vi "Grid_Init_v4.vi"(6 "Part of multigrid":bool, 7 "resume":T1, 8 "Error in":errorcluster, 10 "Settings":T2={"Drift Correction Settings"={"Drift Correction every"=80, "Drift correction Pixels"=256, "Channel index (0-23)"=0, "MaxImagesBack"=2, "Threshold"=2, "Increment"=8, "max applied Drift Correction"=20, "Correct Drift"=TRUE, "Correlate"=0, "Correct z drift"=FALSE, "zdrift \nDuration (s)"=0.0}, "Spectroscopy Setting"={"Imaging Current"=1e-11, "ref Current"=7e-11, "tip Speed (m/s)"=2e-09, "Imaging Bias"=0.02, "ref Bias"=-0.1, "preSTS delay [ms]"=500, "STS z offset"=2e-10, "during Spec Bias (V)"=-0.1, "trigger1 < Hz"=0.0, "trigger 2 >Hz"=0.0, "autoStop"=FALSE, "Spectroscopy"=0, "PLL ON/OFF"=TRUE, "readjust setpoint every "=1, "z Reference"=FALSE, "Lock In"=TRUE}, "Misc"={"File name"="symmetric_node_zOff=200p", "Email when finished"="cornelius.krull@monash.edu,Dhaneesh.Gopalakrishnan@monash.edu,marina.castelli@monash.edu"}, "Grid Settings"={"type"=1, "type order"=1, "X pixel"=0, "Y pixel"=0, "Grid_Parms"={"center X (m)"=0.0, "center Y (m)"=0.0, "width (m)"=0.0, "height (m)"=0.0, "angle (deg)"=0.0}}} {"Grid Settings"."type order" items=["Line", "Grid"]; "Grid Settings"."type" items=["Line", "Grid"]; "Spectroscopy Setting"."Spectroscopy" items=["Bias", "zSpec"]; "Spectroscopy Setting"."trigger 2 >Hz" format="%#_6p"; "Spectroscopy Setting"."trigger1 < Hz" format="%#_6p"; "Spectroscopy Setting"."during Spec Bias (V)" format="%#_5p"; "Spectroscopy Setting"."STS z offset" format="%#_6p"; "Spectroscopy Setting"."ref Bias" format="%#_6p"; "Spectroscopy Setting"."Imaging Bias" format="%#_6p"; "Spectroscopy Setting"."tip Speed (m/s)" format="%.2p"; "Spectroscopy Setting"."ref Current" format="%#_6p"; "Spectroscopy Setting"."Imaging Current" format="%#_6p"; "Drift Correction Settings"."Correlate" items=["first Frame", "successive Frames"]; "Drift Correction Settings"."max applied Drift Correction" min=1 max=100 step=1 format="%.0p"; "Drift Correction Settings"."Threshold" min=1 step=1; "Drift Correction Settings"."Channel index (0-23)" items=["Current"=0, "Z (m)"=14]}, 11 "Application reference":refnum<vi>) -> (0 "error out":errorcluster, 1 "FileRefs":T3, 2 "Settings out":T2={"Drift Correction Settings"={"Drift Correction every"=80, "Drift correction Pixels"=256, "Channel index (0-23)"=0, "MaxImagesBack"=2, "Threshold"=2, "Increment"=8, "max applied Drift Correction"=20, "Correct Drift"=TRUE, "Correlate"=0, "Correct z drift"=FALSE, "zdrift \nDuration (s)"=0.0}, "Spectroscopy Setting"={"Imaging Current"=1e-11, "ref Current"=7e-11, "tip Speed (m/s)"=2e-09, "Imaging Bias"=0.02, "ref Bias"=-0.1, "preSTS delay [ms]"=500, "STS z offset"=2e-10, "during Spec Bias (V)"=-0.1, "trigger1 < Hz"=0.0, "trigger 2 >Hz"=0.0, "autoStop"=FALSE, "Spectroscopy"=0, "PLL ON/OFF"=TRUE, "readjust setpoint every "=1, "z Reference"=FALSE, "Lock In"=TRUE}, "Misc"={"File name"="symmetric_node_zOff=200p", "Email when finished"="cornelius.krull@monash.edu,Dhaneesh.Gopalakrishnan@monash.edu,marina.castelli@monash.edu"}, "Grid Settings"={"type"=1, "type order"=1, "X pixel"=0, "Y pixel"=0, "Grid_Parms"={"center X (m)"=0.0, "center Y (m)"=0.0, "width (m)"=0.0, "height (m)"=0.0, "angle (deg)"=0.0}}} caption="Settings" {"Grid Settings"."type order" items=["Line", "Grid"]; "Grid Settings"."type" items=["Line", "Grid"]; "Spectroscopy Setting"."Spectroscopy" items=["Bias", "zSpec"]; "Spectroscopy Setting"."trigger 2 >Hz" format="%#_6p"; "Spectroscopy Setting"."trigger1 < Hz" format="%#_6p"; "Spectroscopy Setting"."during Spec Bias (V)" format="%#_5p"; "Spectroscopy Setting"."STS z offset" format="%#_6p"; "Spectroscopy Setting"."ref Bias" format="%#_6p"; "Spectroscopy Setting"."Imaging Bias" format="%#_6p"; "Spectroscopy Setting"."tip Speed (m/s)" format="%.2p"; "Spectroscopy Setting"."ref Current" format="%#_6p"; "Spectroscopy Setting"."Imaging Current" format="%#_6p"; "Drift Correction Settings"."Correlate" items=["first Frame", "successive Frames"]; "Drift Correction Settings"."max applied Drift Correction" min=1 max=100 step=1 format="%.0p"; "Drift Correction Settings"."Threshold" min=1 step=1; "Drift Correction Settings"."Channel index (0-23)" items=["Current"=0, "Z (m)"=14]}, 3 "Application ref out":refnum<vi>, 5 "DC images":dbl[][][](array[numeric]))   [LabVIEW 2014]
uses:
  <userlib>/Nanonis Prog Interface V5/Nanonis Prog Interface.lvlib
panel:
  # "RUN smart tilt before starting the GRID\nImg Angle = 0  CHECK CUTOFF\nmove tip to reference point for tip height"
  # "z Spectroscopy"
  # "GRID points"
  # "Increase this if no Drift was detected for \na certain number of images"
  # "% of image size"
  # "RUN smart tilt before starting the GRID\nImg Angle = 0  CHECK CUTOFF\nmove tip to reference point for tip height"
  # "z Spectroscopy"
  # "GRID points"
  # "Increase this if no Drift was detected for \na certain number of images"
  # "% of image size"
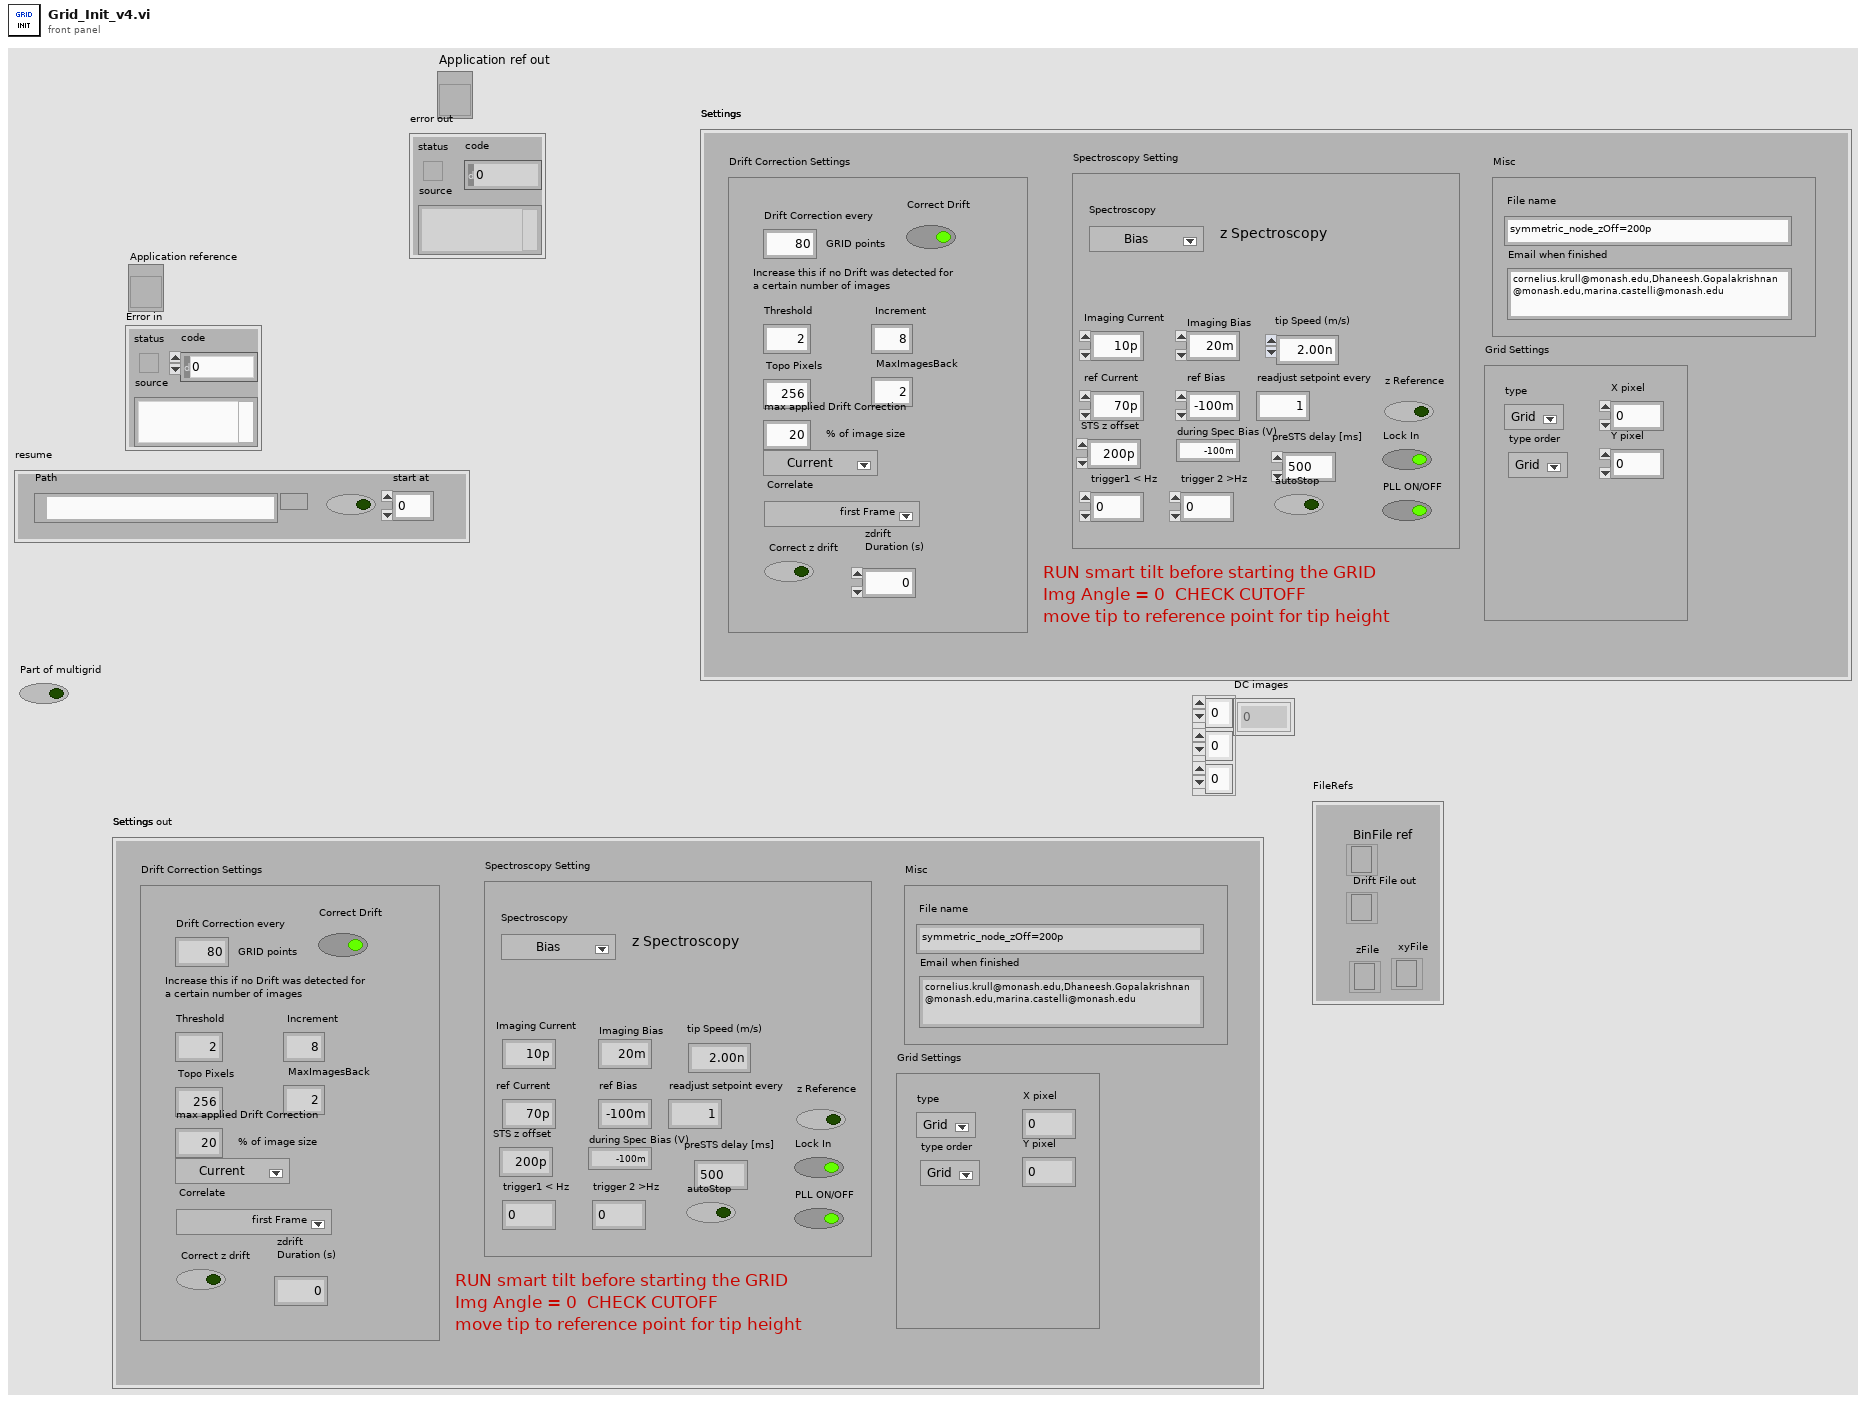
[diagram p1: front panel]
types:
  T1 = cluster{"resume Grid":bool, "Path":path, "start at":i32}
  T2 = cluster{"Drift Correction Settings":cluster{"Drift Correction every":i32, "Drift correction Pixels":i32, "Channel index (0-23)":u8, "MaxImagesBack":i32, "Threshold":i32, "Increment":i32, "max applied Drift Correction":i32, "Correct Drift":bool, "Correlate":u16, "Correct z drift":bool, "zdrift \nDuration (s)":dbl}, "Spectroscopy Setting":cluster{"Imaging Current":dbl, "ref Current":dbl, "tip Speed (m/s)":sgl, "Imaging Bias":dbl, "ref Bias":dbl, "preSTS delay [ms]":u32, "STS z offset":dbl, "during Spec Bias (V)":sgl, "trigger1 < Hz":sgl, "trigger 2 >Hz":sgl, "autoStop":bool, "Spectroscopy":u16, "PLL ON/OFF":bool, "readjust setpoint every ":i32, "z Reference":bool, "Lock In":bool}, "Misc":cluster{"File name":string, "Email when finished":string}, "Grid Settings":cluster{"type":u16, "type order":u16, "X pixel":i32, "Y pixel":i32, "Grid_Parms":cluster{"center X (m)":sgl, "center Y (m)":sgl, "width (m)":sgl, "height (m)":sgl, "angle (deg)":sgl}}}
  T3 = cluster{"Drift File out":refnum<file>, "zFile":refnum<file>, "BinFile ref":refnum<file>, "xyFile":refnum<file>}
  T4 = cluster{"type":u16, "type order":u16, "X pixel":i32, "Y pixel":i32, "Grid_Parms":cluster{"center X (m)":sgl, "center Y (m)":sgl, "width (m)":sgl, "height (m)":sgl, "angle (deg)":sgl}}
  T5 = cluster{"type":u16, "type order":u16, "X pixel":dbl, "Y pixel":dbl, "Grid_Parms":cluster{"center X (m)":sgl, "center Y (m)":sgl, "width (m)":sgl, "height (m)":sgl, "angle (deg)":sgl}}
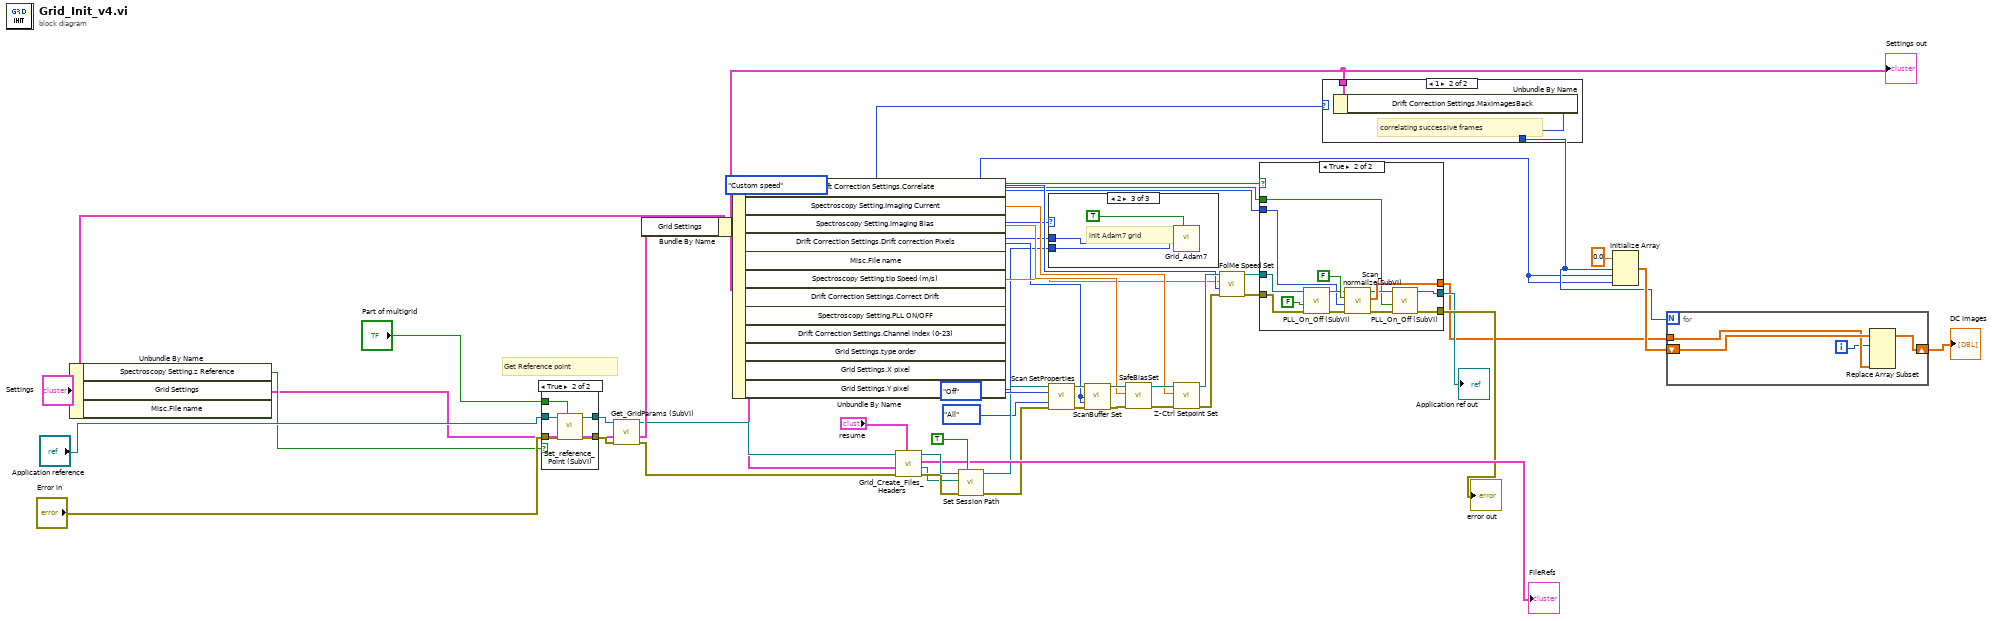
[diagram p0: block diagram]
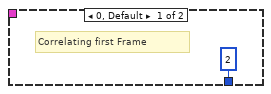
[diagram p4: hidden frame]
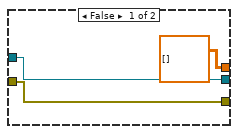
[diagram p5: hidden frame]
diagram:
  # "Get Reference point"
  n1 = Unbundle By Name("Settings") -> ("Spectroscopy Setting.z Reference"=w49:bool, "Grid Settings"=w46:T4)  [unwired: 1 out]
  n2 = case shown="True" w49 {
    tunnel: "Application reference" -> [w53 w58]
    tunnel: "Error in" -> [w52 w57]
    tunnel: [w53 w56] -> w48
    tunnel: [w52 w55] -> w47
    tunnel: "Part of multigrid" -> [_ w54]
    frame False {
    }
    frame True {
      n3 = call "Set_reference_Point (SubVI).vi"("Part of multigrid"=w54, "error in (no error)"=w57, "Application in"=w58) -> ("error out"=w55:errorcluster, "Application out"=w56:refnum<vi>)  [unwired: 7 in]
    }
  }
  n4 = call "Get_GridParams (SubVI).vi"("error in (no error)"=w47, "Grid Settings"=w46, "Application in"=w48) -> ("error out"=w42:errorcluster, "Grid Settings"=w44:T5, "Application out"=w43:refnum<vi>)  [unwired: 5 in, 1 out]
  n5 = Bundle By Name(cluster="Settings", "Grid Settings"=w44) -> (w6:T2)
  "Settings out" <- w6
  n6 = Unbundle By Name(w6) -> ("Drift Correction Settings.Correlate"=w7:u16, "Spectroscopy Setting.Imaging Current"=w26:dbl, "Spectroscopy Setting.Imaging Bias"=w29:dbl, "Drift Correction Settings.Drift correction Pixels"=w8:i32, "Spectroscopy Setting.tip Speed (m/s)"=w22:sgl, "Drift Correction Settings.Correct Drift"=w17:bool, "Spectroscopy Setting.PLL ON/OFF"=w16:bool, "Drift Correction Settings.Channel index (0-23)"=w15:u8, "Grid Settings.type order"=w5:u16, "Grid Settings.X pixel"=w4:i32, "Grid Settings.Y pixel"=w3:i32)  [unwired: 1 out]
  n7 = call "Grid_Create_Files_Headers.vi"("resume"="resume", "Error in (no error)"=w42, "Settings"=w6, "Application ref in"=w43) -> ("error out"=w39:errorcluster, "topoFilePath"=w14:path, "FileRefs"=→"FileRefs":T3, "Application ref out"=w41:refnum<vi>)  [unwired: 4 in]
  n8 = call <userlib>:"Set Session Path.vi"("Save settings to previous? (False)"=TRUE, "error in (no error)"=w39, "Session Folder"=w14, "Application ref in"=w41) -> ("error out"=w33:errorcluster, "Application ref out"=w34:refnum<vi>)  [unwired: 6 in]
  n9 = case shown="2" w5 {
    tunnel: w4 -> [_ _ w60]
    tunnel: w3 -> [_ _ w59]
    frame 0, Default {
    }
    frame 1 {
    }
    frame 2 {
      # "init Adam7 grid"
      n10 = call "Grid_Adam7.vi"("reset"=TRUE, "py 2"=w59, "px 2"=w60) -> ()  [unwired: 7 in, 2 out]
    }
  }
  n11 = call <userlib>:"Scan SetProperties.vi"("Application ref in"=w34, "Continuous scan"=enum16{"No change", "On", "Off"}."Off", "Auto save"=enum16{"No change", "All", "Next", "Off"}."All", "Error in (no error)"=w33) -> ("Application ref out"=w36:refnum<vi>, "Error out"=w35:errorcluster)  [unwired: 10 in]
  n12 = call <userlib>:"ScanBuffer Set.vi"("Application ref in"=w36, "Pixels"=w8, "Lines"=w8, "error in (no error)"=w35) -> ("Application ref out"=w31:refnum<vi>, "error out"=w30:errorcluster)  [unwired: 10 in]
  n13 = call "SafeBiasSet.vi"("Application ref in"=w31, "Bias (V)"=w29, "error in (no error)"=w30) -> ("Application ref out"=w27:refnum<vi>, "Error out"=w28:errorcluster)  [unwired: 6 in]
  n14 = call <userlib>:"Z-Ctrl Setpoint Set.vi"("error in (no error)"=w28, "Z Controller setpoint"=w26, "Application ref in"=w27) -> ("error out"=w24:errorcluster, "Application ref out"=w25:refnum<vi>)  [unwired: 7 in]
  n15 = call <userlib>:"FolMe Speed Set.vi"("error in (no error)"=w24, "Speed Setting (Custom)"=enum32{"Scan speed", "Custom speed"}."Custom speed", "Speed (m/s)"=w22, "Application ref in"=w25) -> ("error out"=w20:errorcluster, "Application ref out"=w21:refnum<vi>)  [unwired: 4 in]
  n16 = case shown="True" w17 {
    tunnel: [dbl[][] [] ("Array") w77] -> w11
    tunnel: w21 -> [w64 w75]
    tunnel: [w64 w71] -> w18
    tunnel: w20 -> [w62 w70]
    tunnel: [w62 w67] -> w19
    tunnel: w16 -> [_ w66]
    tunnel: w15 -> [_ w65]
    frame False {
    }
    frame True {
      n17 = call "PLL_On_Off (SubVI).vi"("error in (no error)"=w70, "Output ON/OFF (F=OFF)"=FALSE, "Application in"=w75) -> ("error out"=w69:errorcluster, "Application out"=w74:refnum<vi>)  [unwired: 7 in]
      n18 = call "Scan_normailze(SubVI).vi"("error in (no error)"=w69, "Channel index (0-23)"=w65, "Normalization"=FALSE ("Boolean"), "Application in"=w74) -> ("error out"=w68:errorcluster, "Array"=w77:dbl[][], "Application out"=w72:refnum<vi>)  [unwired: 5 in]
      n19 = call "PLL_On_Off (SubVI).vi"("error in (no error)"=w68, "Output ON/OFF (F=OFF)"=w66, "Application in"=w72) -> ("error out"=w67:errorcluster, "Application out"=w71:refnum<vi>)  [unwired: 7 in]
    }
  }
  "Application ref out" <- w18
  "error out" <- w19
  n20 = case shown="1" w7 {
    tunnel: w6 -> [_ w80]
    tunnel: [2 ("MaxImagesBack") w79] -> w10
    frame 0, Default {
      # "Correlating first Frame"
    }
    frame 1 {
      # "correlating successive frames"
      n21 = Unbundle By Name(w80) -> ("Drift Correction Settings.MaxImagesBack"=w79:i32)
    }
  }
  n22 = Initialize Array(0.0 ("element"), w10, w8, w8) -> (w12:dbl[][][])
  n23 = for {
    N: w10 -> [_]
    tunnel: w11 -> [w83]
    shift-right: [w82] -> w9
    shift-left: w12 -> [w84]
    i -> [w81]
    n24 = Replace Array Subset(array=w84, new element=w83, index (dim 0)=w81) -> (w82:dbl[][][])  [unwired: 2 in]
  }
  "DC images" <- w9
